vi "Prepare Monkeys from Notes.vi"(0 "Monkey Business Notes":string[](array[string]), 1 "Bored Operation":string="/ 3") -> (2 "LCD":u64, 3 "Monkeys":T1)   [LabVIEW 2020, in "AoC 2022.lvlib"]
uses:
  AoC 2022.lvlib
  Monkey.ctl
  Monkeys.ctl
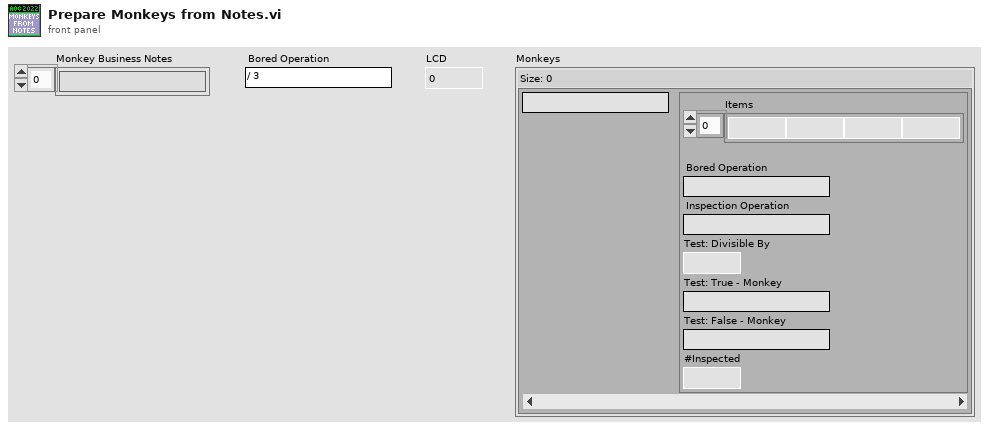
[diagram p1: front panel]
types:
  T1 = typedef "AoC 2022.lvlib/Monkeys.ctl" = map{string, T2}
  T2 = typedef "AoC 2022.lvlib/Monkey.ctl" = cluster{"Items":u64[], "Bored Operation":string, "Inspection Operation":string, "Test: Divisible By":u64, "Test: True - Monkey":string, "Test: False - Monkey":string, "#Inspected":i32}
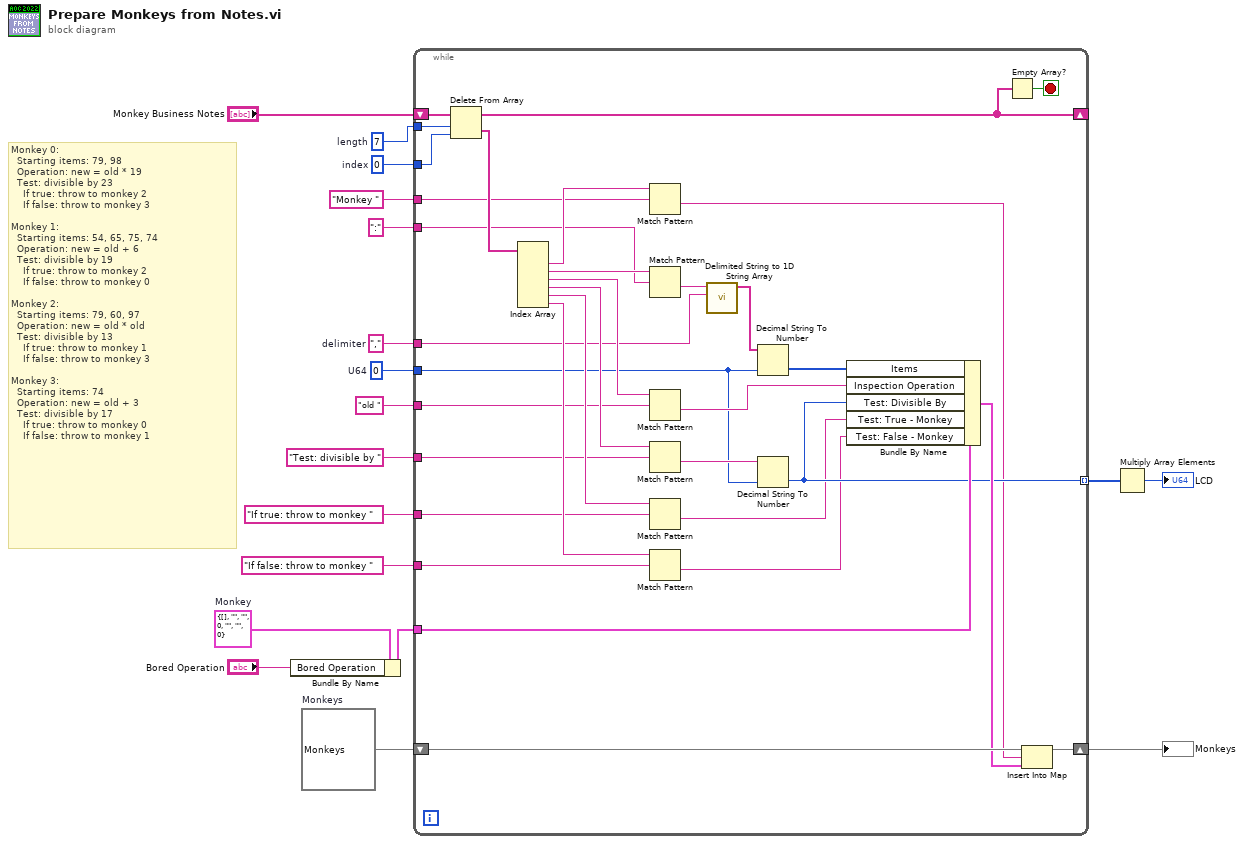
[diagram p0: block diagram]
diagram:
  w4 = u64 0  # U64
  w9 = ","  # delimiter
  w17 = T2 {"Items"=[], "Bored Operation"="", "Inspection Operation"="", "Test: Divisible By"=0, "Test: True - Monkey"="", "Test: False - Monkey"="", "#Inspected"=0}  # Monkey
  w16 = T1 {}  # Monkeys
  w15 = 0  # index
  w14 = 7  # length
  # "Monkey 0:\n  Starting items: 79, 98\n  Operation: new = old * 19\n  Test: divisible by 23\n    If true: throw to monkey 2\n    If false: throw to monkey 3\n\nMonkey 1:\n  Starting items: 54, 65, 75, 74\n  Operation: new = old + 6\n  Test: divisible by 19\n    If true: throw to monkey 2\n    If false: throw to monkey 0\n\nMonkey 2:\n  Starting items: 79, 60, 97\n  Operation: new = old * old\n  Test: divisible by 13\n    If true: throw to monkey 1\n    If false: throw to monkey 3\n\nMonkey 3:\n  Starting items: 74\n  Operation: new = old + 3\n  Test: divisible by 17\n    If true: throw to monkey 0\n    If false: throw to monkey 1"
  n1 = Bundle By Name(cluster=w17, "Bored Operation"="Bored Operation") -> (w6:T2)
  n2 = while {
    tunnel: w14 -> [w50]
    tunnel: w15 -> [w49]
    shift-right: [w47] -> _
    shift-left: "Monkey Business Notes" -> [w51]
    shift-right: [w44] -> w2
    shift-left: w16 -> [w45]
    tunnel: w6 -> [w43]
    tunnel: "old " -> [w31]
    tunnel: "Test: divisible by " -> [w30]
    tunnel: "If false: throw to monkey " -> [w29]
    tunnel: "If true: throw to monkey " -> [w28]
    tunnel: w9 -> [w27]
    tunnel: ":" -> [w26]
    tunnel: "Monkey " -> [w25]
    tunnel: w4 -> [w22]
    tunnel: [w23] -> w3 mode=indexing
    stop <- w48 stop-if-true
    n3 = Delete From Array(array=w51, length=w50, index=w49) -> (deleted portion=w46:string[], array with subset deleted=w47:string[])
    n4 = Index Array(array=w46) -> (element #1=w32:string, element #2=w41:string, element #3=w37:string, element #4=w35:string, element #5=w34:string, element #6=w33:string)  [unwired: 6 in]
    n5 = Match Pattern(string=w32, regular expression=w25) -> (after substring=w21:string)  [unwired: 1 in, 3 out]
    n6 = Match Pattern(string=w41, regular expression=w26) -> (after substring=w40:string)  [unwired: 1 in, 3 out]
    n7 = Match Pattern(string=w37, regular expression=w31) -> (after substring=w36:string)  [unwired: 1 in, 3 out]
    n8 = Match Pattern(string=w35, regular expression=w30) -> (after substring=w24:string)  [unwired: 1 in, 3 out]
    n9 = Match Pattern(string=w34, regular expression=w28) -> (after substring=w20:string)  [unwired: 1 in, 3 out]
    n10 = Match Pattern(string=w33, regular expression=w29) -> (after substring=w19:string)  [unwired: 1 in, 3 out]
    n11 = call <vilib>:"Delimited String to 1D String Array.vi"("delimiter"=w27, "delimited string"=w40) -> ("string array"=w39:string[])  [unwired: 9 in]
    n12 = Decimal String To Number(string=w39, default (0L)=w22) -> (number=w38:u64[])  [unwired: 1 in, 1 out]
    n13 = Decimal String To Number(string=w24, default (0L)=w22) -> (number=w23:u64)  [unwired: 1 in, 1 out]
    n14 = Bundle By Name(cluster=w43, "Items"=w38, "Inspection Operation"=w36, "Test: Divisible By"=w23, "Test: True - Monkey"=w20, "Test: False - Monkey"=w19) -> (w42:T2)
    n15 = Empty Array?(array=w47) -> (empty?=w48:bool)
    n16 = Insert Into Map(map in=w45, key=w21, value=w42) -> (map out=w44:T1)  [unwired: 2 out]
  }
  "Monkeys" <- w2
  n17 = Multiply Array Elements(1:w3) -> (0:→"LCD":u64)
